vi "FP_Get Primary Monitor Workspace.vi"(10 "Primary":T3, 11 "All Work Spaces":T2=[{"Bounds"={"Left"=-10, "Top"=0, "Right"=0, "Bottom"=-10}, "Depth"=0}, {"Bounds"={"Left"=0, "Top"=0, "Right"=10, "Bottom"=10}, "Depth"=0}, {"Bounds"={"Left"=-10, "Top"=-10, "Right"=0, "Bottom"=0}, "Depth"=0}, {"Bounds"={"Left"=0, "Top"=-10, "Right"=10, "Bottom"=0}, "Depth"=0}, {"Bounds"={"Left"=10, "Top"=-10, "Right"=20, "Bottom"=0}, "Depth"=0}, {"Bounds"={"Left"=10, "Top"=0, "Right"=20, "Bottom"=10}, "Depth"=0}, {"Bounds"={"Left"=-10, "Top"=10, "Right"=0, "Bottom"=20}, "Depth"=0}, {"Bounds"={"Left"=0, "Top"=10, "Right"=10, "Bottom"=20}, "Depth"=0}, {"Bounds"={"Left"=10, "Top"=10, "Right"=20, "Bottom"=20}, "Depth"=0}]) -> (2 "Index Out":i32, 3 "Primary Work Space Out":T1)   [LabVIEW 2025]
uses:
  <vilib>/Utility/miscctls.llb/LVRectTypeDef.ctl
  <vilib>/Utility/miscctls.llb/LVAllMonitorsDisplayTypeDef.ctl
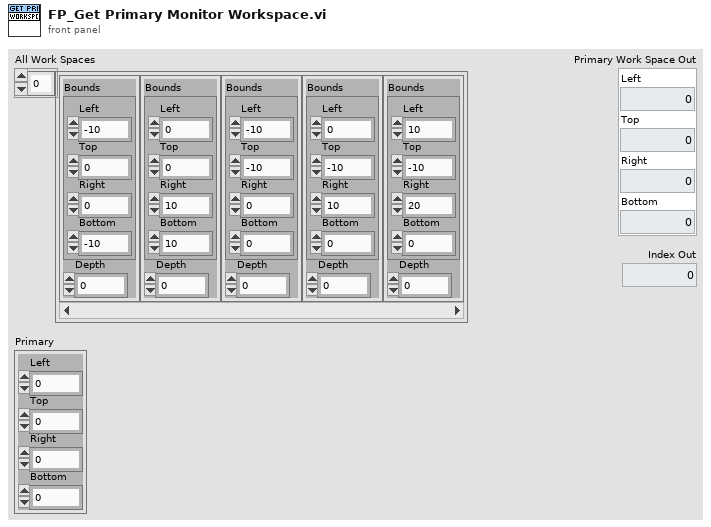
[diagram p1: front panel]
types:
  T1 = cluster{"Left":i16, "Top":i16, "Right":i16, "Bottom":i16}
  T2 = typedef "LVAllMonitorsDisplayTypeDef.ctl" = cluster{"Bounds":cluster{"Left":i16, "Top":i16, "Right":i16, "Bottom":i16}, "Depth":i16}[]
  T3 = typedef "LVRectTypeDef.ctl" = cluster{"Left":i16, "Top":i16, "Right":i16, "Bottom":i16}
  T4 = cluster{"Left":bool, "Top":bool, "Right":bool, "Bottom":bool}
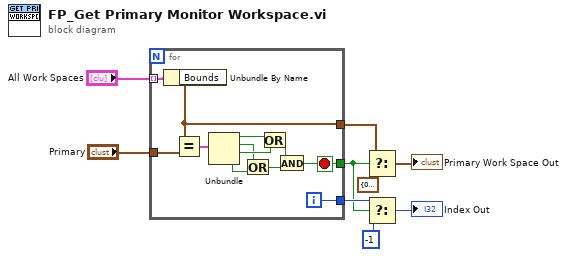
[diagram p0: block diagram]
diagram:
  n1 = for {
    tunnel: "All Work Spaces" -> [w21] mode=indexing
    tunnel: "Primary" -> [w20]
    tunnel: [w12] -> w6
    tunnel: [w11] -> w3
    tunnel: [w10] -> w7
    i -> [w10]
    stop <- w11 stop-if-true
    n2 = Unbundle By Name(w21) -> ("Bounds"=w12:T1)
    n3 = Equal?(x=w12, y=w20) -> (x = y?=w19:T4)
    n4 = Unbundle(w19) -> ("Left"=w18:bool, "Top"=w16:bool, "Right"=w17:bool, "Bottom"=w15:bool)
    n5 = Or(x=w16, y=w15) -> (x .or. y?=w14:bool)
    n6 = Or(x=w18, y=w17) -> (x .or. y?=w13:bool)
    n7 = And(x=w13, y=w14) -> (x .and. y?=w11:bool)
  }
  n8 = Select(t=w6, s=w3, f=T1 {"Left"=0, "Top"=0, "Right"=0, "Bottom"=0}) -> (s? t:f=→"Primary Work Space Out":T1)
  n9 = Select(t=w7, s=w3, f=-1) -> (s? t:f=→"Index Out":i32)
